vi "Backup and Self Correct Rx Offset.vi"(0 "niUsrpRio session":T1={"FPGA Interface"=refnum, "RIO Interface Number"=0, "Data Clock Rate"=0, "FPGA Data Clock Rate"=0, "Global Settings Register Bus"=refnum, "Radio 0 Settings Register Bus"=refnum, "Radio 1 Settings Register Bus"=refnum, "Radio Settings Bus Semaphore"=refnum, "DB Queues"=[], "Characterization Data Valid?"=FALSE, "EEPROM Header"={"Checksum"=0, "Product Code"=0, "Hardware Current Version"=0, "Hardware Oldest Compatible Version"=0, "EEPROM Map Current Version"=0, "EEPROM Map Oldest Compatible Version"=0, "User Password"="", "Pointer to Factory Header"=0, "Pointer to User Header"=0, "Recommended Interval"=0, "Number of Reserved Bytes"=9, "Number of Daughterboards"=0, "Daughterboard IDs"=[], "Daughterboard Serial Numbers"=[]}, "Device Data Header"={"Checksum"=0, "Number of Channels"=0, "Number of Gain Settings"=[], "Pointer to Characterization Data"=[], "Number of Reserved Bytes"=27, "Number of Frequencies"=[]}, "EEPROM Characterization Header"={"Checksum"=0, "Date"=timestamp(0 s since 1904-01-01), "Temperature"=0.0, "Misc. Info"="", "Pointer to Device Data Header"=0, "Number of Reserved Bytes"=28}, "Characterization Data"=[], "FPGA Current Version"=0, "FPGA Oldest Compatible Version"=0, "Fixed Logic Current Version"=0, "Fixed Logic Oldest Compatible Version"=0, "FPGA Radio Settings Bus Current Version"=0, "FPGA Radio Settings Bus Oldest Compatible Version"=0, "FPGA Board Config Current Version"=0, "FPGA Board Config Oldest Compatible Version"=0, "Daughterboard Clock Rate"=0, "daughterboard configuration session handles"=[]} {"Daughterboard Clock Rate" format="%#.3pHz"; "FPGA Data Clock Rate" format="%#.3pHz"; "Data Clock Rate" format="%#.3pHz"; "Characterization Data"."Frequencies [Hz]" format="%#_6p"; "EEPROM Characterization Header"."Pointer to Device Data Header" format="%x"; "EEPROM Characterization Header"."Checksum" format="%x"; "Device Data Header"."Pointer to Characterization Data" format="%x"; "Device Data Header"."Checksum" format="%x"; "EEPROM Header"."Pointer to User Header" format="%x"; "EEPROM Header"."Pointer to Factory Header" format="%x"; "EEPROM Header"."Product Code" format="%x"; "EEPROM Header"."Checksum" format="%x"}, 5 "channel to update":i32(ring) items=["Rx 0", "Tx 0", "Rx 1", "Tx 1"], 7 "tuning settle (ms)":u32=100, 9 "backup existing data?":bool=TRUE, 11 "Error In":errorcluster, 12 "prompt for backup file path?":bool=TRUE, 13 "backup folder path":path) -> (4 "niUsrpRio session (out)":T1={"FPGA Interface"=refnum, "RIO Interface Number"=0, "Data Clock Rate"=0, "FPGA Data Clock Rate"=0, "Global Settings Register Bus"=refnum, "Radio 0 Settings Register Bus"=refnum, "Radio 1 Settings Register Bus"=refnum, "Radio Settings Bus Semaphore"=refnum, "DB Queues"=[], "Characterization Data Valid?"=FALSE, "EEPROM Header"={"Checksum"=0, "Product Code"=0, "Hardware Current Version"=0, "Hardware Oldest Compatible Version"=0, "EEPROM Map Current Version"=0, "EEPROM Map Oldest Compatible Version"=0, "User Password"="", "Pointer to Factory Header"=0, "Pointer to User Header"=0, "Recommended Interval"=0, "Number of Reserved Bytes"=9, "Number of Daughterboards"=0, "Daughterboard IDs"=[], "Daughterboard Serial Numbers"=[]}, "Device Data Header"={"Checksum"=0, "Number of Channels"=0, "Number of Gain Settings"=[], "Pointer to Characterization Data"=[], "Number of Reserved Bytes"=27, "Number of Frequencies"=[]}, "EEPROM Characterization Header"={"Checksum"=0, "Date"=timestamp(0 s since 1904-01-01), "Temperature"=0.0, "Misc. Info"="", "Pointer to Device Data Header"=0, "Number of Reserved Bytes"=28}, "Characterization Data"=[], "FPGA Current Version"=0, "FPGA Oldest Compatible Version"=0, "Fixed Logic Current Version"=0, "Fixed Logic Oldest Compatible Version"=0, "FPGA Radio Settings Bus Current Version"=0, "FPGA Radio Settings Bus Oldest Compatible Version"=0, "FPGA Board Config Current Version"=0, "FPGA Board Config Oldest Compatible Version"=0, "Daughterboard Clock Rate"=0, "daughterboard configuration session handles"=[]} {"Daughterboard Clock Rate" format="%#.3pHz"; "FPGA Data Clock Rate" format="%#.3pHz"; "Data Clock Rate" format="%#.3pHz"; "Characterization Data"."Frequencies [Hz]" format="%#_6p"; "EEPROM Characterization Header"."Pointer to Device Data Header" format="%x"; "EEPROM Characterization Header"."Checksum" format="%x"; "Device Data Header"."Pointer to Characterization Data" format="%x"; "Device Data Header"."Checksum" format="%x"; "EEPROM Header"."Pointer to User Header" format="%x"; "EEPROM Header"."Pointer to Factory Header" format="%x"; "EEPROM Header"."Product Code" format="%x"; "EEPROM Header"."Checksum" format="%x"}, 6 "Updated Characterization Data":T8[](array[typedef]) {"Frequencies [Hz]" format="%#_6p"}, 15 "Error Out":errorcluster)   [LabVIEW 2021]
uses:
  <instrlib>/niUsrpRio/Config/v1/Host/Public/EEPROM Header.ctl
  <instrlib>/niUsrpRio/Config/v1/Host/Public/EEPROM Device Data Header.ctl
  <instrlib>/niUsrpRio/Config/v1/Host/Public/EEPROM Characterization Header.ctl
  <instrlib>/niUsrpRio/Config/v1/Host/Public/Characterization Data.ctl
  <instrlib>/niUsrpRio/Config/v1/Host/Public/IQ Imbalance.ctl
  <instrlib>/niUsrpRio/Config/v1/Host/Public/niUsrpRio Session.ctl
  <instrlib>/_niInstr/Register Bus/v0/Host/Public/Register Bus Session.ctl
  <instrlib>/_niInstr/Register Bus/v0/Host/Private/Session Data.ctl
  <instrlib>/niUsrpRio/Config/v1/Host/Private/DB Queue Reference.ctl
  <instrlib>/niUsrpRio/Config/v1/Host/Private/Daughterboard Data.ctl
  <instrlib>/niUsrpRio/Config/v1/Host/Private/ATR state data.ctl
  <instrlib>/niUsrpRio/Config/v1/Host/Private/Antenna Configuration.ctl
  <instrlib>/niUsrpRio/Config/v1/Host/Private/CPLD Power Mode.ctl
  <vilib>/Utility/error.llb/Error Cluster From Error Code.vi
  <vilib>/Utility/file.llb/Write Delimited Spreadsheet (DBL).vi
  <vilib>/ErrorRing/Error Ring.xnode
  <instrlib>/niUsrpRio/Config/v1/Host/niUsrpRio Config v1 Host.lvlib
  <instrlib>/_niInstr/Register Bus/v0/Host/niInstr Register Bus v0 Host.lvlib
panel:
  out "Original Characterization Data":T8[](array[typedef]) {"Frequencies [Hz]" format="%#_6p"}
  out "EEPROM Characterization Header":T7={"Checksum"=0, "Date"=timestamp(0 s since 1904-01-01), "Temperature"=0.0, "Misc. Info"="", "Pointer to Device Data Header"=0, "Number of Reserved Bytes"=28} {"Pointer to Device Data Header" format="%x"; "Checksum" format="%x"}
  out "Device Data Header":T6={"Checksum"=0, "Number of Channels"=0, "Number of Gain Settings"=[], "Pointer to Characterization Data"=[], "Number of Reserved Bytes"=27, "Number of Frequencies"=[]} {"Pointer to Characterization Data" format="%x"; "Checksum" format="%x"}
  out "EEPROM Header":T5={"Checksum"=0, "Product Code"=0, "Hardware Current Version"=0, "Hardware Oldest Compatible Version"=0, "EEPROM Map Current Version"=0, "EEPROM Map Oldest Compatible Version"=0, "User Password"="", "Pointer to Factory Header"=0, "Pointer to User Header"=0, "Recommended Interval"=0, "Number of Reserved Bytes"=9, "Number of Daughterboards"=0, "Daughterboard IDs"=[], "Daughterboard Serial Numbers"=[]} {"Pointer to User Header" format="%x"; "Pointer to Factory Header" format="%x"; "Product Code" format="%x"; "Checksum" format="%x"}
  out "Characterization Data Valid?":bool
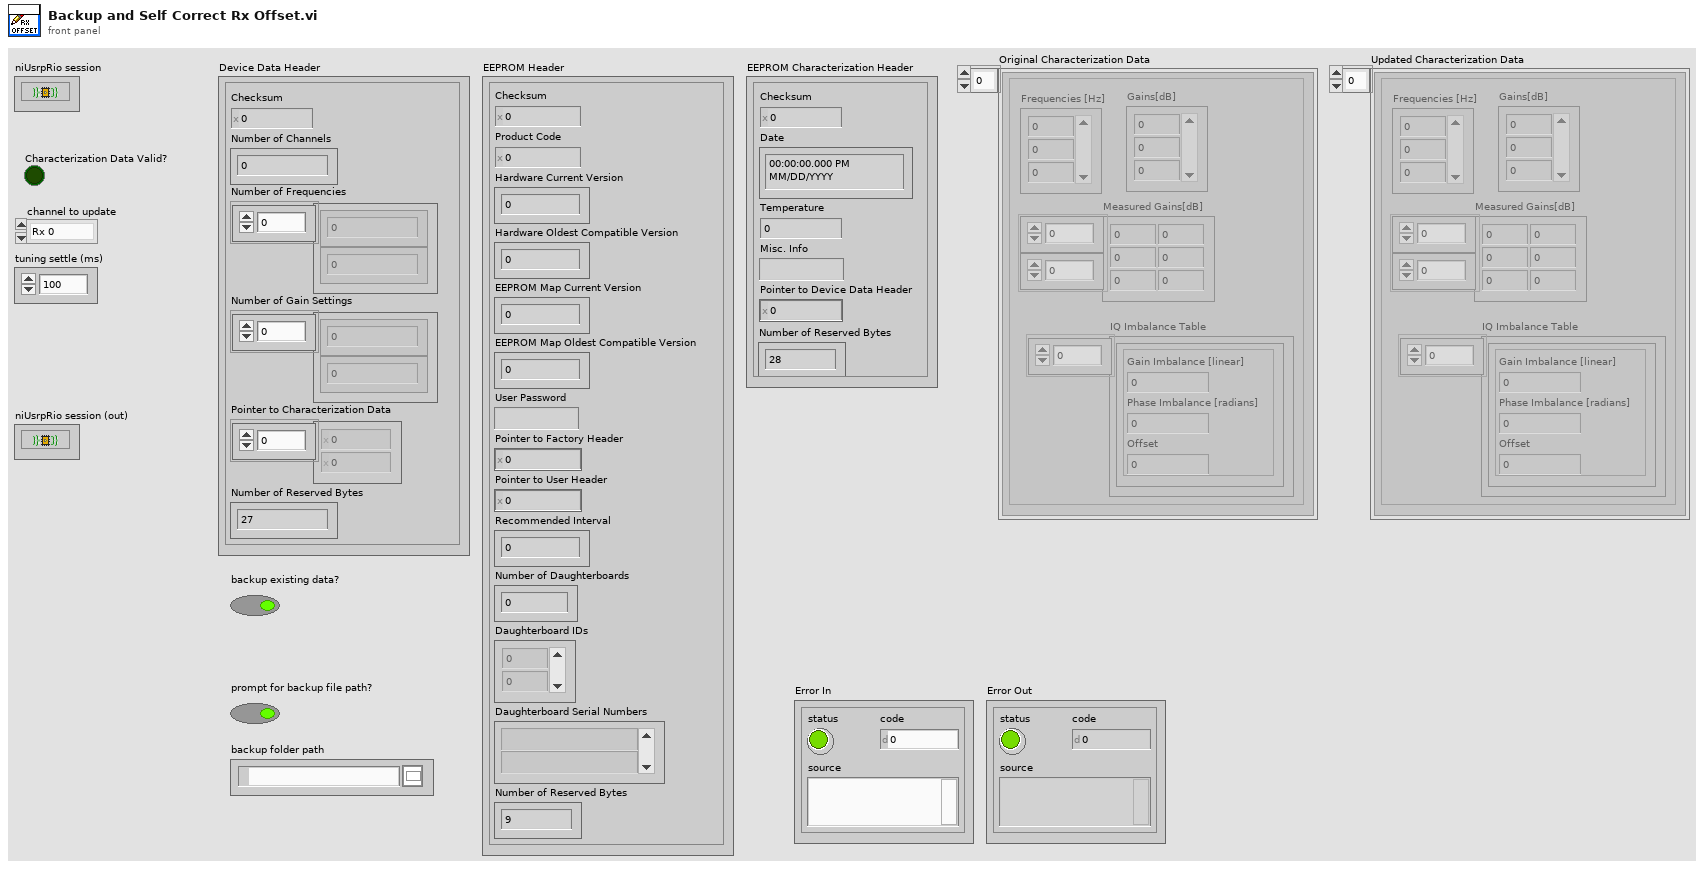
[diagram p1: front panel]
types:
  T1 = typedef "niUsrpRio Config v1 Host.lvlib/niUsrpRio Session.ctl" = cluster{"FPGA Interface":refnum<k20>, "RIO Interface Number":u32, "Data Clock Rate":u32, "FPGA Data Clock Rate":u32, "Global Settings Register Bus":T2, "Radio 0 Settings Register Bus":T2, "Radio 1 Settings Register Bus":T2, "Radio Settings Bus Semaphore":T3, "DB Queues":T4[], "Characterization Data Valid?":bool, "EEPROM Header":T5, "Device Data Header":T6, "EEPROM Characterization Header":T7, "Characterization Data":T8[], "FPGA Current Version":u32, "FPGA Oldest Compatible Version":u32, "Fixed Logic Current Version":u32, "Fixed Logic Oldest Compatible Version":u32, "FPGA Radio Settings Bus Current Version":u32, "FPGA Radio Settings Bus Oldest Compatible Version":u32, "FPGA Board Config Current Version":u32, "FPGA Board Config Oldest Compatible Version":u32, "Daughterboard Clock Rate":u32, "daughterboard configuration session handles":u64[]}
  T2 = typedef "niInstr Register Bus v0 Host.lvlib/Register Bus Session.ctl" = refnum<queue>
  T3 = typedef "Semaphore RefNum" = refnum<k1>
  T4 = typedef "niUsrpRio Config v1 Host.lvlib/DB Queue Reference.ctl" = refnum<queue>
  T5 = typedef "niUsrpRio Config v1 Host.lvlib/EEPROM Header.ctl" = cluster{"Checksum":u32, "Product Code":u16, "Hardware Current Version":u16, "Hardware Oldest Compatible Version":u16, "EEPROM Map Current Version":u16, "EEPROM Map Oldest Compatible Version":u16, "User Password":string, "Pointer to Factory Header":u32, "Pointer to User Header":u32, "Recommended Interval":u16, "Number of Reserved Bytes":i32, "Number of Daughterboards":u8, "Daughterboard IDs":u16[], "Daughterboard Serial Numbers":string[]}
  T6 = typedef "niUsrpRio Config v1 Host.lvlib/EEPROM Device Data Header.ctl" = cluster{"Checksum":u32, "Number of Channels":u8, "Number of Gain Settings":u16[], "Pointer to Characterization Data":u32[], "Number of Reserved Bytes":i32, "Number of Frequencies":u16[]}
  T7 = typedef "niUsrpRio Config v1 Host.lvlib/EEPROM Characterization Header.ctl" = cluster{"Checksum":u32, "Date":timestamp, "Temperature":sgl, "Misc. Info":string, "Pointer to Device Data Header":u32, "Number of Reserved Bytes":i32}
  T8 = typedef "niUsrpRio Config v1 Host.lvlib/Characterization Data.ctl" = cluster{"Gains[dB]":dbl[], "Frequencies [Hz]":dbl[], "IQ Imbalance Table":T9[], "Measured Gains[dB]":dbl[][]}
  T9 = typedef "niUsrpRio Config v1 Host.lvlib/IQ Imbalance.ctl" = cluster{"Gain Imbalance [linear]":dbl, "Phase Imbalance [radians]":dbl, "Offset":cdb}
  T10 = typedef "niUsrpRio Config v1 Host.lvlib/DB Types.ctl" = enum16{"sbx", "cbx", "wbx", "unknown", "ubx", "twinrx"}
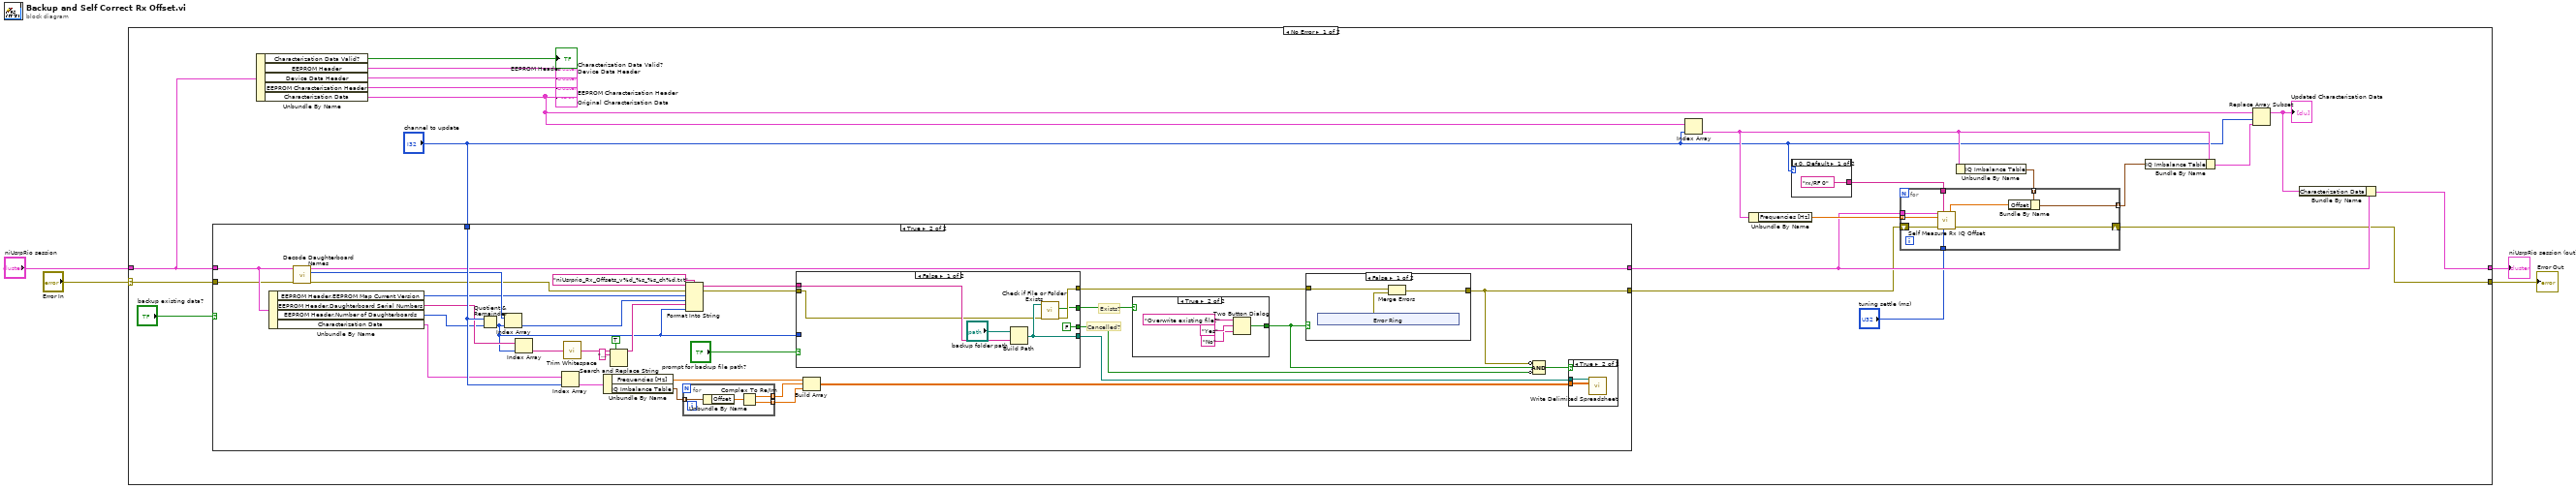
[diagram p0: block diagram]
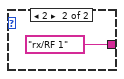
[diagram p2: hidden frame]
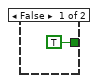
[diagram p5: hidden frame]
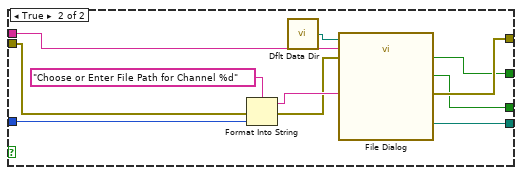
[diagram p6: hidden frame]
diagram:
  n1 = case shown="No Error" "Error In" {
    selector: "Error In" -> [w18 w112]
    tunnel: [w8 w112] -> w4
    tunnel: "niUsrpRio session" -> [w19 w111]
    tunnel: [w20 w111] -> w1
    frame No Error {
      n2 = case shown="True" "backup existing data?" {
        tunnel: w19 -> [w38 w72]
        tunnel: w18 -> [w37 w71]
        tunnel: "channel to update" -> [_ w70]
        tunnel: [w38 w69] -> w13
        tunnel: [w37 w39] -> w12
        frame False {
        }
        frame True {
          # "Cancelled?"
          # "Exists?"
          n3 = Unbundle By Name(w72) -> ("EEPROM Header.EEPROM Map Current Version"=w63:u16, "EEPROM Header.Daughterboard Serial Numbers"=w67:string[], "EEPROM Header.Number of Daughterboards"=w65:u8, "Characterization Data"=w60:T8[])
          n4 = call <instrlib>:"Decode Daughterboard Names.vi"("niUsrpRio Session"=w72, "error in"=w71) -> ("niUsrpRio Session (out)"=w69:T1, "daughterboard names"=w66:T10[], "error out"=w61:errorcluster)  [unwired: 10 in, 1 out]
          n5 = Quotient & Remainder(x=w70, y=w65) -> (floor(x/y)=w44:i32)  [unwired: 1 out]
          n6 = Index Array(array=w66, index=w44) -> (element=w64:T10)
          n7 = Index Array(array=w67, index=w44) -> (element=w55:string)
          n8 = Index Array(array=w60, index=w70) -> (element=w59:T8)
          n9 = call <vilib>:"Trim Whitespace.vi"("string"=w55) -> ("trimmed string"=w54:string)  [unwired: 1 in]
          n10 = Unbundle By Name(w59) -> ("Frequencies [Hz]"=w58:dbl[], "IQ Imbalance Table"=w42:T9[])
          n11 = Search and Replace String(replace all?=TRUE ("replace all? (F)"), input string=w54, search string="\u0000") -> (result string=w51:string)  [unwired: 5 in, 3 out]
          n12 = for {
            tunnel: w42 -> [w76] mode=indexing
            tunnel: [w74] -> w41 mode=indexing
            tunnel: [w73] -> w40 mode=indexing
            n13 = Unbundle By Name(w76) -> ("Offset"=w75:cdb)
            n14 = Complex To Re/Im(x + iy=w75) -> (x=w74:dbl, y=w73:dbl)
          }
          n15 = Format Into String(format string="niUsrprio_Rx_Offsets_v%d_%s_%s_ch%d.txt", error in=w61, w63, w64, w51, w44) -> (resulting string=w62:string, error out=w43:errorcluster)  [unwired: 1 in]
          n16 = case shown="False" "prompt for backup file path?" {
            tunnel: [w94 w108] -> w45
            tunnel: w62 -> [w96 w107]
            tunnel: [w95 w106] -> w56
            tunnel: [FALSE ("cancelled") w105] -> w48
            tunnel: [w93 w103] -> w49
            tunnel: w44 -> [_ w101]
            tunnel: w43 -> [w91 w99]
            frame False {
              n17 = Build Path(base path="backup folder path", name or relative path=w96) -> (appended path=w95:path)
              n18 = call <vilib>:"Check if File or Folder Exists.vi"("error in (no error)"=w91, "path"=w95) -> ("error out"=w94:errorcluster, "file or folder exists?"=w93:bool)  [unwired: 7 in, 1 out]
            }
            frame True {
              n19 = Format Into String(format string="Choose or Enter File Path for Channel %d" ("prompt"), error in=w99, w101) -> (resulting string=w100:string, error out=w98:errorcluster)  [unwired: 1 in]
              n20 = call <vilib>:"Dflt Data Dir.vi"() -> ("App:Default Data Directory"=w104:path)
              n21 = call "File Dialog"("start path"=w104, "prompt"=w100, "default name"=w107, "error in"=w98) -> ("selected path"=w106:path, "exists"=w103:bool, "cancelled"=w105:bool, "error out"=w108:errorcluster)  [unwired: 8 in]
            }
          }
          n22 = Build Array(w58, w41, w40) -> (w57:dbl[][])
          n23 = case shown="True" w49 {
            tunnel: [TRUE ("T button?") w87] -> w46
            frame False {
            }
            frame True {
              n24 = Two Button Dialog(message="Overwrite existing file?", 1:"No" ("F button name (\"Cancel\")"), 2:"Yes" ("T button name (\"OK\")")) -> (T button?=w87:bool)
            }
          }
          n25 = case shown="False" w46 {
            tunnel: w45 -> [w79 w85]
            tunnel: [w77 w85] -> w39
            frame False {
              n26 = xnode "Error Ring"() -> ("error out"=w78:errorcluster)
              n27 = Merge Errors(w79, w78) -> (w77:errorcluster)
            }
            frame True {
            }
          }
          n28 = Compound Arithmetic op=AND(invert w39, w46, invert w48) -> (w47:bool)
          n29 = case shown="True" w47 {
            tunnel: w57 -> [_ w109]
            tunnel: w56 -> [_ w110]
            frame False {
            }
            frame True {
              n30 = call-poly <vilib>:"Write Delimited Spreadsheet.vi"("file path (dialog if empty)"=w110, "2D data"=w109) -> ()  [unwired: 12 in, 2 out]
            }
          }
        }
      }
      n31 = Unbundle By Name(w19) -> ("Characterization Data Valid?"=→"Characterization Data Valid?":bool, "EEPROM Header"=→"EEPROM Header":T5, "Device Data Header"=→"Device Data Header":T6, "EEPROM Characterization Header"=→"EEPROM Characterization Header":T7, "Characterization Data"=w14:T8[])
      "Original Characterization Data" <- w14
      n32 = Index Array(array=w14, index="channel to update") -> (element=w11:T8)
      n33 = Unbundle By Name(w11) -> ("Frequencies [Hz]"=w15:dbl[])
      n34 = case shown="0, Default" "channel to update" {
        tunnel: ["rx/RF 0" ("channel") "rx/RF 1" ("channel")] -> w5
        frame 0, Default {
        }
        frame 2 {
        }
      }
      n35 = Unbundle By Name(w11) -> ("IQ Imbalance Table"=w10:T9[])
      n36 = for {
        tunnel: w5 -> [w36]
        tunnel: w15 -> [w35] mode=indexing
        tunnel: w13 -> [w34]
        shift-right: [w32] -> w8
        shift-left: w12 -> [w33]
        tunnel: w10 -> [w31] mode=indexing
        tunnel: [w29] -> w9 mode=indexing
        tunnel: "tuning settle (ms)" -> [w28]
        n37 = call "Self Measure Rx IQ Offset.vi"("niUsrpRio Session"=w34, "channel"=w36, "carrier freq"=w35, "error in"=w33, "tuning settle (ms)"=w28) -> ("offset"=w30:cdb, "error out"=w32:errorcluster)  [unwired: 7 in, 2 out]
        n38 = Bundle By Name(cluster=w31, "Offset"=w30) -> (w29:T9)
      }
      n39 = Bundle By Name(cluster=w11, "IQ Imbalance Table"=w9) -> (w24:T8)
      n40 = Replace Array Subset(array=w14, new element=w24, index="channel to update") -> (w23:T8[])
      "Updated Characterization Data" <- w23
      n41 = Bundle By Name(cluster=w13, "Characterization Data"=w23) -> (w20:T1)
    }
    frame Error {
    }
  }
  "Error Out" <- w4
  "niUsrpRio session (out)" <- w1
